vi "POS_Query.vi"(0 "System no.":i32=1 min=1 max=4 step=1, 2 "Axes to query":string[](array[string]), 3 "All axes?":bool, 4 "Axis identifier?":bool=TRUE, 5 "error in":errorcluster) -> (14 "Position":dbl[](array[numeric]) format="%.6f", 19 "error out":errorcluster)   [LabVIEW 2020]
doc: "GCS 3.0\n=====\n\nPOS? (Get Real Position)\n\nDescription\nQueries the current position of the axes.\n\nFormat\nPOS?[ <AxisID>]\n\nArguments\nPOS? without arguments queries all axes of the controller.\n<AxisID>\nAn axis of the controller\nThe available axes can be queried with USG? SYS.\nPossible values: Alias of the axis (p. 94) \n\nResponse\n{<AxisID>\"=\"<CurrentPosition>LF}\n<CurrentPosition>\nCurrent position of the axis in physical units\nThe data format is float.\nPossible values: Dependent on the axis\n\nExample\nThe physical unit for axes 1 and 2 is queried using the SPV? command (p. 63), and then the \ncurrent position is queried - firstly for all available axes and then only for axis 1.\n>>spv? ram AXIS_1 - 0x106\n<<RAM AXIS_1 - 0x106=mm\n>>spv? ram AXIS_2 - 0x106\n<<RAM AXIS_2 - 0x106=mm\n>>pos?\n<<AXIS_1=0.0\n<<AXIS_2=0.0\n>>pos? axis_1\n<<AXIS_1=0.0\n\nNotes\nThe physical unit for the axis can be queried with the SPV? command via the following \nparameter:\nAXIS_n - 0x106 STRING32 - USR USR - - Configuration Physical Unit Of Position - - \n\nUser command level\nUSR\n\n\nGCS 2.0\n=====\n\nReturns position information (actual or target position, depending on system).\n\nC-880K005: VI only supported when called through PI_Multix.vi\n\nE-516: If All axes? = TRUE, then Axis identifier? must be TRUE\n\nE-710: If All axes? = TRUE, then Axis identifier? must be TRUE . \n\nE-755: If All axes? = TRUE, then Axis identifier? can be FALSE. Command not available for E-755.101.\n\nE-816: All axes? = FALSE, only one axis per command allowed.\n\nC-887, F-206: If All axes? = TRUE, then Axis identifier? can be FALSE. For GCS syntax version = GCS 1.0 (check with CSV?.vi. If CSV?.vi is not supported, syntax version is GCS 1.0), returned position value is the commanded target position for the axis.\n\nC-887, M-8X0: If All axes? = TRUE, then Axis identifier? can be FALSE. For GCS syntax version = GCS 1.0 (check with CSV?.vi. If CSV?.vi is not supported, syntax version is GCS 1.0), returned position value is the commanded target position for the axis.\n\nAll other systems: If All axes? = TRUE, then Axis identifier? can be FALSE."
panel:
  # "POS? (Get Real Position)\n\nQueries the current position of the axes."
  # "Query"
  # "If all axes: use"
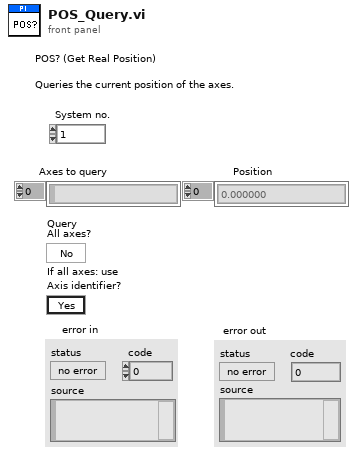
[diagram p1: front panel]
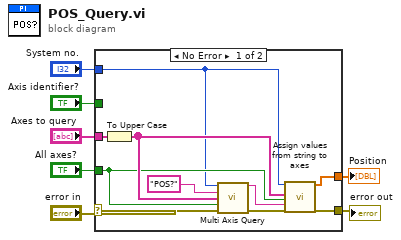
[diagram p0: block diagram]
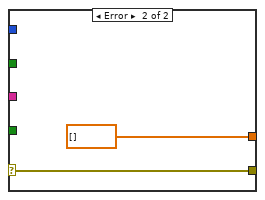
[diagram p2: hidden frame]
diagram:
  n1 = case shown="No Error" "error in" {
    selector: "error in" -> [w16 w19]
    tunnel: [w11 dbl[] [] ("Values")] -> w3
    tunnel: "Axes to query" -> [w17 _]
    tunnel: [w13 w19] -> w4
    tunnel: "System no." -> [w8 _]
    tunnel: "All axes?" -> [w9 _]
    tunnel: "Axis identifier?" -> [_ _]
    frame No Error {
      n2 = To Upper Case(1:w17) -> (0:w12:string[])
      n3 = call "Multi Axis Query.vi"("System no."=w8, "Command"="POS?", "Axis"=w12, "All axes?"=w9, "error in (no error)"=w16) -> ("Answer"=w10:string, "error out"=w14:errorcluster)  [unwired: 9 in]
      n4 = call "Assign values from string to axes.vi"("System no."=w8, "Queried axes"=w12, "All axes queried?"=w9, "Input String"=w10, "error in"=w14) -> ("Values"=w11:dbl[], "error out"=w13:errorcluster)  [unwired: 4 in, 9 out]
    }
    frame Error {
      (unwired) string[] [] ("Axes to query out")
    }
  }
  "error out" <- w4
  "Position" <- w3
